vi "MRC Acquire.vi"(8 "error in (no error)":errorcluster, 9 "Message Data":variant, 10 "MRC notifier":refnum<notifier>, 11 "Hardware Resources in":T1={"MFC Definition"={"MFC Port"="", "MFC Enable"=TRUE, "Baud Rate"=0, "Interface type"=enum."RS-485", "Address"=0}, "Set Point Options"={"Setpoint Value"=0.0, "Mass Flow EU 2"="", "Setpoint Source"="", "Valve Mode"=""}, "Writer Queue"=refnum, "Enable"=FALSE, "Update Rate"=0, "MRC Chamber Enable"=FALSE, "Selected Gas"="", "Address String"=""} {"Set Point Options"."Setpoint Value" min=0.0 max=0.62495 format="%.5f"}) -> (0 "error out":errorcluster, 1 "Message Data Out":variant)   [LabVIEW 2020, in "MRC Module.lvlib"]
doc: "Perform the acquisition. Replace the contents of this diagram with calls to acquisition hardware."
uses:
  MRC Module.lvlib
  MRC Configuration.ctl
  support/Message Queue/Message Cluster.ctl
  support/Message Queue/Message Queue.lvlib
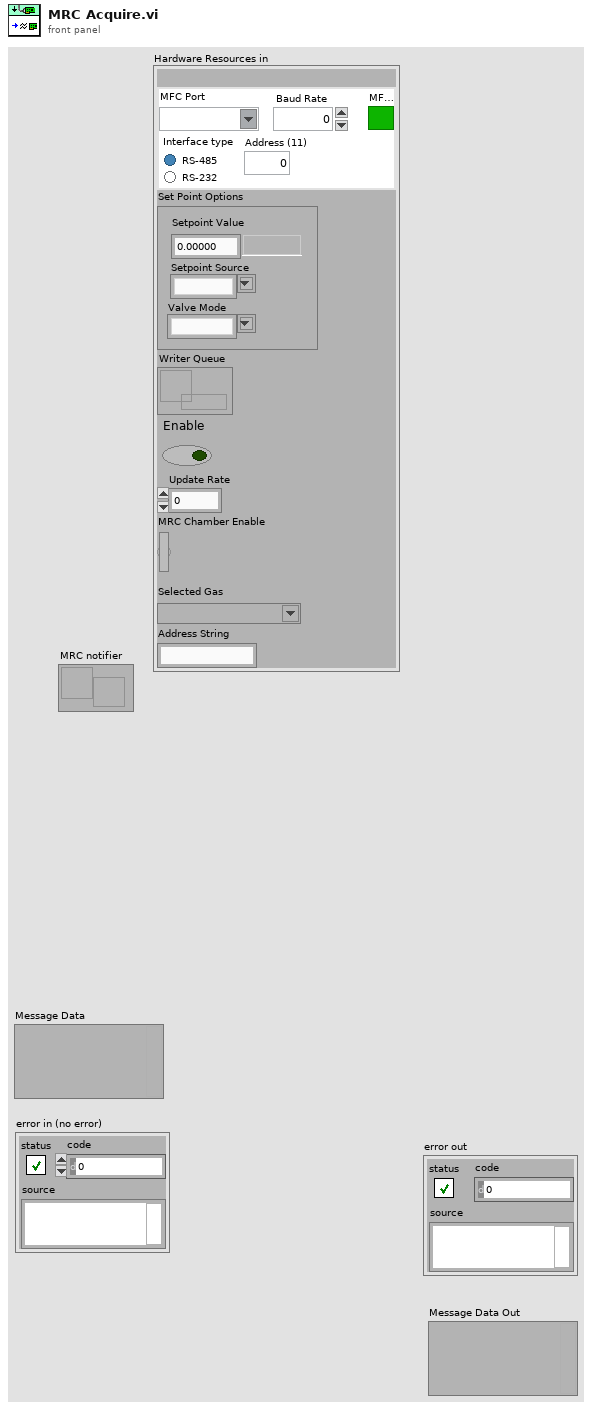
[diagram p1: front panel]
types:
  T1 = typedef "MRC Module.lvlib/MRC Configuration.ctl" = cluster{"MFC Definition":cluster{"MFC Port":refnum<visa-resource-name>, "MFC Enable":bool, "Baud Rate":i32, "Interface type":enum32{"RS-485", "RS-232"}, "Address":i32}, "Set Point Options":cluster{"Setpoint Value":dbl, "Mass Flow EU 2":string, "Setpoint Source":string, "Valve Mode":string}, "Writer Queue":refnum<queue>, "Enable":bool, "Update Rate":u32, "MRC Chamber Enable":bool, "Selected Gas":string, "Address String":string}
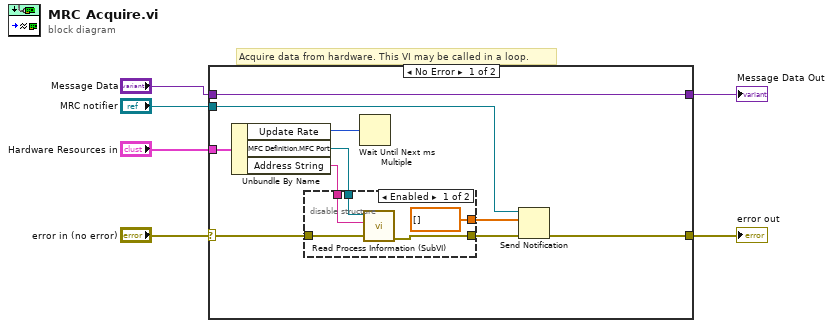
[diagram p0: block diagram]
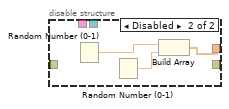
[diagram p2: hidden frame]
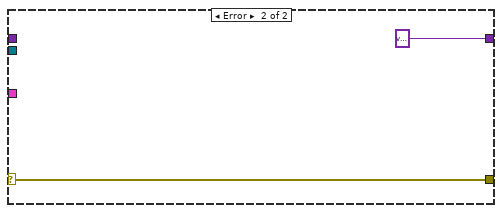
[diagram p3: hidden frame]
diagram:
  # "Acquire data from hardware. This VI may be called in a loop."
  n1 = case shown="No Error" "error in (no error)" {
    selector: "error in (no error)" -> [w11 w26]
    tunnel: [w16 w26] -> w5
    tunnel: [w13 variant ("Message Data Out")] -> w4
    tunnel: "Message Data" -> [w13 _]
    tunnel: "Hardware Resources in" -> [w15 _]
    tunnel: "MRC notifier" -> [w14 _]
    frame No Error {
      n2 = Unbundle By Name(w15) -> ("Update Rate"=w12:u32, "MFC Definition.MFC Port"=w10:refnum<visa-resource-name>, "Address String"=w7:string)
      n3 = disable-structure shown="Enabled" {
        disable-tunnel: w11 -> [w21 _]
        disable-tunnel: w10 -> [w19 _]
        disable-tunnel: [w20 _] -> w9
        disable-tunnel: [dbl[] [] w22] -> w8
        disable-tunnel: w7 -> [w17 _]
        frame Enabled {
          n4 = call "Read Process Information (SubVI).vi"("error in (no error)"=w21, "Address"=w17, "VISA Refnum in"=w19) -> ("error out"=w20:errorcluster)  [unwired: 4 in, 4 out]
        }
        frame Disabled {
          n5 = Random Number (0-1)() -> (number: 0 to 1=w24:dbl)
          n6 = Random Number (0-1)() -> (number: 0 to 1=w23:dbl)
          n7 = Build Array(w24, w23) -> (w22:dbl[])
        }
      }
      n8 = Wait Until Next ms Multiple(millisecond multiple=w12) -> ()  [unwired: 1 out]
      n9 = Send Notification(notification=w8, notifier=w14, error in (no error)=w9) -> (error out=w16:errorcluster)  [unwired: 1 out]
    }
    frame Error {
    }
  }
  "error out" <- w5
  "Message Data Out" <- w4
